vi "Timer FGV.vi"(7 "Action":T1, 8 "error in (no error)":errorcluster) -> (0 "error out":errorcluster, 3 "Elapsed Time":dbl)   [LabVIEW 2015]
uses:
  Timer Actions.ctl
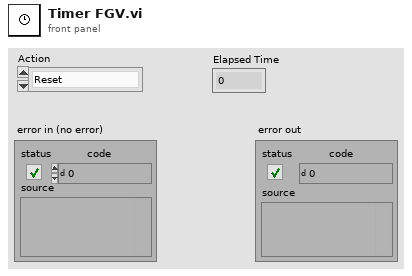
[diagram p1: front panel]
types:
  T1 = typedef "Timer Actions.ctl" = enum16{"Reset", "Get"}
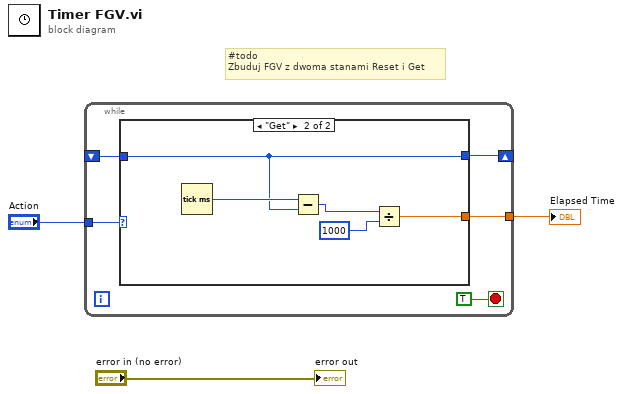
[diagram p0: block diagram]
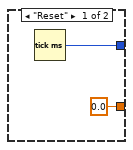
[diagram p2: hidden frame]
diagram:
  # "#todo \nZbuduj FGV z dwoma stanami Reset i Get"
  n1 = while {
    shift-right: [w5] -> _
    shift-left: _ -> [w4]
    tunnel: "Action" -> [w7]
    tunnel: [w6] -> w1
    stop <- TRUE stop-if-true
    n2 = case shown="\"Get\"" w7 {
      tunnel: [0.0 w12] -> w6
      tunnel: [w9 w11] -> w5
      tunnel: w4 -> [_ w11]
      frame "Reset" {
        n3 = Tick Count (ms)() -> (millisecond timer value=w9:u32)
      }
      frame "Get" {
        n4 = Tick Count (ms)() -> (millisecond timer value=w15:u32)
        n5 = Subtract(x=w15, y=w11) -> (x-y=w14:u32)
        n6 = Divide(x=w14, y=u32 1000) -> (x/y=w12:dbl)
      }
    }
  }
  "Elapsed Time" <- w1
  "error out" <- "error in (no error)"
